vi "FPGA_MapDIOChannelEnumToModuleLine.vi"(11 "DIOChannel":T1) -> (2 "ActualDIOBitMask(U32)":u32 format="%.0b", 3 "ActualDIOChannel(U8)":u8)   [LabVIEW 2017]
uses:
  <vilib>/Rock Robotics/SystemInterfaces/DIO/FPGA_DIOChannel.ctl
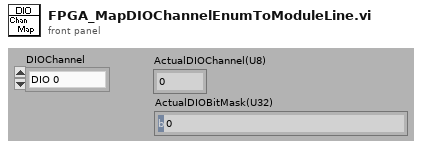
[diagram p1: front panel]
types:
  T1 = typedef "FPGA_DIOChannel.ctl" = enum8{"DIO 0", "DIO 1", "DIO 2", "DIO 3", "DIO 4", "DIO 5", "DIO 6", "DIO 7", "DIO 8", "DIO 9", "DIO MXP 0", "DIO MXP 1", "DIO MXP 2", "DIO MXP 3", "DIO MXP 4", "DIO MXP 5", "DIO MXP 6", "DIO MXP 7", "DIO MXP 8", "DIO MXP 9", "DIO MXP 10", "DIO MXP 11", "DIO MXP 12", "DIO MXP 13", "DIO MXP 14", "DIO MXP 15", "SPI Port CS1", "SPI Port CS2", "SPI Port CS3", "SPI Port MISO", "SPI Port MOSI", "Invalid"}
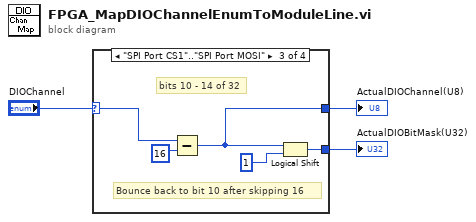
[diagram p0: block diagram]
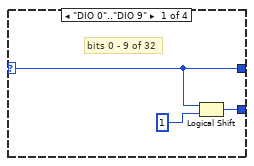
[diagram p2: hidden frame]
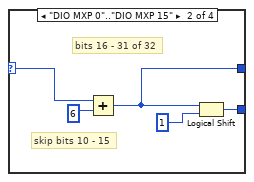
[diagram p3: hidden frame]
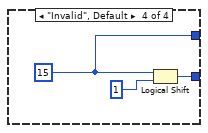
[diagram p4: hidden frame]
diagram:
  n1 = case shown="\"SPI Port CS1\"..\"SPI Port MOSI\"" "DIOChannel" {
    selector: "DIOChannel" -> [w4 w8 w13 _]
    tunnel: [w4 w7 w12 w17] -> w3
    tunnel: [w5 w10 w15 w18] -> w2
    frame "DIO 0".."DIO 9" {
      # "bits 0 - 9 of 32"
      n2 = Logical Shift(y=w4, x=u16 1 ("Value")) -> (x << y=w5:u16)
    }
    frame "DIO MXP 0".."DIO MXP 15" {
      # "skip bits 10 - 15"
      # "bits 16 - 31 of 32"
      n3 = Add(x=w8, y=u8 6) -> (x+y=w7:u8)
      n4 = Logical Shift(y=w7, x=u32 1 ("Value")) -> (x << y=w10:u32)
    }
    frame "SPI Port CS1".."SPI Port MOSI" {
      # "Bounce back to bit 10 after skipping 16"
      # "bits 10 - 14 of 32"
      n5 = Subtract(x=w13, y=u8 16) -> (x-y=w12:u8)
      n6 = Logical Shift(y=w12, x=u32 1 ("Value")) -> (x << y=w15:u32)
    }
    frame "Invalid", Default {
      w17 = u8 15 ("x+y")
      n7 = Logical Shift(y=w17, x=u32 1 ("Value")) -> (x << y=w18:u32)
    }
  }
  "ActualDIOChannel(U8)" <- w3
  "ActualDIOBitMask(U32)" <- w2
